vi "TestFindString.vi"() -> ()   [LabVIEW 2014]
panel:
  out "resulting string":string
  out "output 1":dbl
  out "offset past match":i32
  out "after substring":string
  out "before substring":string
  out "match substring":string
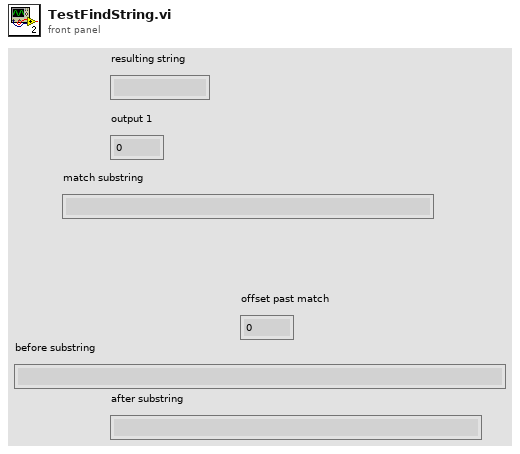
[diagram p1: front panel]
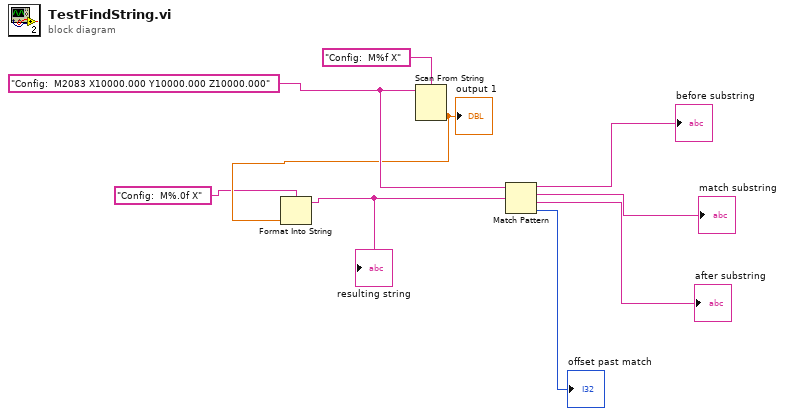
[diagram p0: block diagram]
diagram:
  w4 = "Config:  M2083 X10000.000 Y10000.000 Z10000.000" ("string")
  n1 = Scan From String(format string="Config:  M%f X", input string=w4) -> (output 1=w3:dbl)  [unwired: 3 in, 3 out]
  "output 1" <- w3
  n2 = Format Into String(format string="Config:  M%.0f X" ("regular expression"), w3) -> (resulting string=w2:string)  [unwired: 2 in, 1 out]
  "resulting string" <- w2
  n3 = Match Pattern(string=w4, regular expression=w2) -> (before substring=→"before substring":string, match substring=→"match substring":string, after substring=→"after substring":string, offset past match=→"offset past match":i32)  [unwired: 1 in]
